vi "BNC555.destructor.vi"(0 "i ref in":refnum<vi>, 5 "error in":errorcluster) -> (19 "error out":errorcluster)   [LabVIEW 2014, in "BNC555.lvlib"]
doc: "This is the destructor of a class.\n\nLicense Agreement for this software:\n\nCopyright (C)\nGesellschaft für Schwerionenforschung, GSI\nPlanckstr. 1\n64291 Darmstadt\nGermany\n\nContact: D.Beck@gsi.de \n\nThis program is free software; you can redistribute it and/or modify it under the terms of the \nGNU General Public License as published by the Free Software Foundation; either version 2 of \nthe license, or (at your option) any later version.\n\nThis program is distributed in the hope that it will be useful, but WITHOUT ANY WARRANTY; \nwithout even the implied warranty of MERCHANTABILITY or FITNESS FOR A PARTICULAR PURPOSE. See the GNU General License for more details (http://www.gnu.org).\n\nGesellschaft für Schwerionenforschung, GSI\nPlanckstr. 1, 64291 Darmstadt, Germany\nFor all questions and ideas contact: M.Richter@gsi.de, H.Brand@gsi.de or D.Beck@gsi.de.\nLast update: 16-JUN-2004"
uses:
  BNC555.lvlib
  CS_PHELIX/PH_Basics/PH_PSDBWriter/PH_PSDBWriter.lvlib
  CSlibraries-extern/DimLVEvent/LVDimInterface/LVDimInterface.lvlib
  CS_PHELIX/PH_Basics/PH_StatusHandler/PH_StatusHandler.lvlib
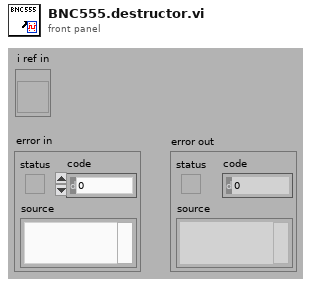
[diagram p1: front panel]
types:
  T1 = typedef "BNC555.lvlib/BNC555.i attribute.ctl" = cluster{"Information":cluster{"VISA resource name":refnum<visa-resource-name>, "Baud Rate (1:9600)":u16}, "Channel Array":T2[], "System":T3, "GUI Refs":cluster{"Delete":refnum<vi>, "Information":refnum<vi>, "System":refnum<vi>, "Channel Array":refnum<vi>, "Device Error":refnum<vi>, "Instr Driver Revision":refnum<vi>, "Instr Firmware Revision":refnum<vi>, "Instr Option":refnum<vi>, "Self-Test Response":refnum<vi>}, "Service IDs Channelinfo":i32[], "Service ID T0 Mode":i32}
  T2 = typedef "BNC555 - Driver np.lvlib/BNC555 All Chan Parameters.ctl" = cluster{"Chan #":i32, "Chan State":bool, "Chan Delay":dbl, "Chan Width":dbl, "Chan Mode":enum16{"Normal", "Single", "Burst", "Divide by N"}, "Chan Burst #":u32, "Chan Divide #":u32, "Chan Pol Out":enum16{"Normal", "Complement", "Inverted"}, "Chan Level Out":enum16{"TTL", "Adjustable", "35 Volt"}, "Chan Lev Adjust":dbl, "Chan Gate Pol":enum16{"Normal", "Complement", "Inverted"}, "Chan Gate State":bool}
  T3 = typedef "BNC555 - Driver np.lvlib/BNC555 All Sys Parameters.ctl" = cluster{"Sys Period":dbl, "Sys Oscillator":bool, "Sys Mode":enum16{"Normal", "Single", "Burst", "Duty Cycle"}, "Sys Burst #":u32, "Sys DC On":u32, "Sys DC Off":u32, "Sys Trig Mode":enum16{"Disabled", "Triggered", "Gated"}, "Sys Trig Lev":dbl, "Sys Gate State":bool, "Sys Trig Edge":bool, "Sys State":bool}
  T4 = enum16{"SetAttribute", "GetAttribute", "CreateAttribute", "DestroyAttribute", "DestroyAllAtributes"}
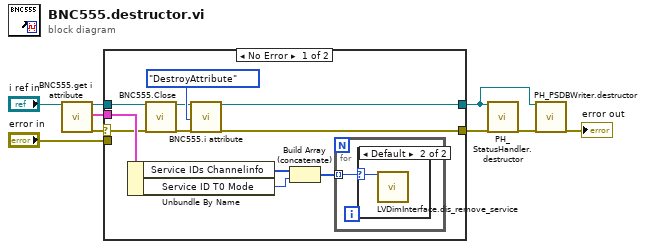
[diagram p0: block diagram]
diagram:
  n1 = call "BNC555.get i attribute.vi"("i ref in"="i ref in") -> ("i ref out"=w8:refnum<vi>, "i attribute"=w7:T1, "error out"=w2:errorcluster)  [unwired: 16 in]
  n2 = case shown="No Error" w2 {
    selector: w2 -> [w10 _]
    tunnel: [w19 w24] -> w9
    tunnel: w8 -> [w18 w23]
    tunnel: w7 -> [w17 _]
    tunnel: [w11 w23] -> w3
    tunnel: "error in" -> [_ w24]
    frame No Error {
      n3 = Unbundle By Name(w17) -> ("Service IDs Channelinfo"=w16:i32[], "Service ID T0 Mode"=w14:i32)
      n4 = call "BNC555.Close.vi"("i ref in"=w18, "error in (no error)"=w10) -> ("i ref out"=w13:refnum<vi>, "error out"=w12:errorcluster)  [unwired: 16 in]
      n5 = call "BNC555.i attribute.vi"("VI Refnum"=w13, "Action"=T4."DestroyAttribute", "error in (no error)"=w12) -> ("VI Refnum out"=w11:refnum<vi>, "error out"=w19:errorcluster)  [unwired: 14 in, 1 out]
      n6 = Build Array (concatenate)(w16, w14) -> (w15:i32[])
      n7 = for {
        tunnel: w15 -> [w21] mode=indexing
        n8 = case shown="Default" w21 {
          selector: w21 -> [_ w22]
          frame -1 {
          }
          frame Default {
            n9 = call "LVDimInterface.dis_remove_service.vi"("my_serviceID"=w22) -> ()  [unwired: 18 in, 1 out]
          }
        }
      }
    }
    frame Error {
    }
  }
  n10 = call "PH_StatusHandler.destructor.vi"("i ref in"=w3, "error in(no error)"=w9) -> ("error out"=w4:errorcluster)  [unwired: 17 in]
  n11 = call "PH_PSDBWriter.destructor.vi"("i ref in"=w3, "error in(no error)"=w4) -> ("error out"=→"error out":errorcluster)  [unwired: 17 in]
